vi "Launch Topic Actor Core.vi"(8 "error in (no error)":errorcluster, 9 "Inbox":refnum<class "Message Transport Queue.lvclass">, 10 "Topic Name":string, 11 "Topic Actor in":refnum<class "Topic Actor.lvclass">) -> (0 "error out":errorcluster)   [LabVIEW 2016, in "Stream Mediator.lvlib" / "Topic Actor.lvclass"]
doc: "--\nCopyright © 2017 Composed SystemsI All rights reserved.\n\nAuthor: Jon McBee <jon.mcbee@composed.io>\n\nThis library is provided \"AS IS\" ,WITHOUT WARRANTIES OR\nCONDITIONS OF ANY KIND, either express or implied.\n\nComposed Systems -- composed.io\n\nStream 0.0.1.1\nJon McBee - Composed Systems\nCopyright (c) 2017, Composed Systems"
uses:
  <userlib>/Composed Systems/Stream/Mediator/Classes/Topic Actor/Topic Actor.lvclass
  <userlib>/Composed Systems/Stream/Mediator/Classes/Message Transport Queue/Message Transport Queue.lvclass
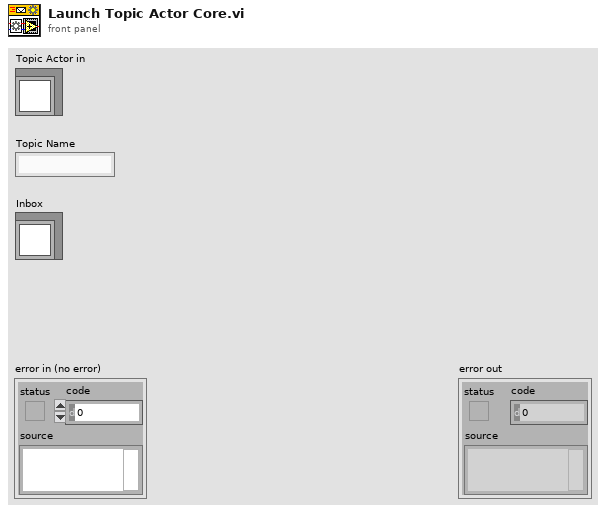
[diagram p1: front panel]
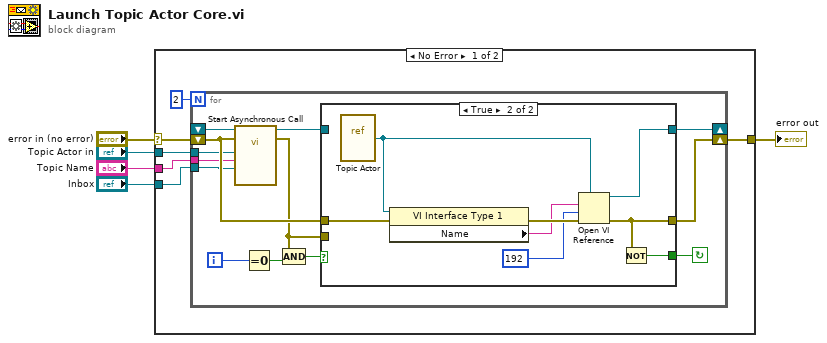
[diagram p0: block diagram]
diagram:
  n1 = case shown="No Error" "error in (no error)" {
    selector: "error in (no error)" -> [w10 w35]
    tunnel: [w9 w35] -> w4
    tunnel: "Topic Actor in" -> [w8 _]
    tunnel: "Topic Name" -> [w7 _]
    tunnel: "Inbox" -> [w6 _]
    frame No Error {
      n2 = for {
        N: 2 -> [_]
        shift-right: [w24] -> w9
        shift-left: w10 -> [w20]
        shift-right: [w22] -> _
        shift-left: _ -> [w21]
        tunnel: w8 -> [w14]
        tunnel: w7 -> [w13]
        tunnel: w6 -> [w12]
        i -> [w17]
        stop <- w23 continue-if-true
        n3 = call-by-ref "Start Asynchronous Call"(reference=w21, error in=w20, "Inbox"=w12, "Topic Name"=w13, "Topic Actor in"=w14) -> (reference out=w15:refnum<vi>, error out=w16:errorcluster)  [unwired: 9 in]
        n4 = Equal To 0?(x=w17) -> (x = 0?=w18:bool)
        n5 = Compound Arithmetic op=AND(w16, w18) -> (w19:bool)
        n6 = case shown="True" w19 {
          tunnel: w20 -> [_ w34]
          tunnel: [w26 w29] -> w24
          tunnel: [_ w28] -> w23
          tunnel: [w25 w27] -> w22
          tunnel: w16 -> [w26 _]
          tunnel: w15 -> [w25 _]
          frame False {
          }
          frame True {
            n7 = vi-ref <userlib>:"Topic Actor.vi"() -> (w32:refnum<vi>)
            n8 = property class="VI Interface Type 1"(reference=w32, error in=w34) -> (error out=w33:errorcluster, "Name"=w31:string)  [unwired: 1 out]
            n9 = Open VI Reference(type specifier VI Refnum (for type only)=w32, vi path=w31, options=192, error in (no error)=w33) -> (vi reference=w27:refnum<vi>, error out=w29:errorcluster)  [unwired: 2 in]
            n10 = Not(x=w29) -> (.not. x?=w28:bool)
          }
        }
      }
    }
    frame Error {
    }
  }
  "error out" <- w4
